vi "Menu.Simulate, Set Menu State.vi"(8 "error in (no error)":errorcluster, 9 "Sim Enable":bool, 10 "Menu Tag":string, 11 "Menu Ref":refnum<k9>) -> (0 "error out":errorcluster, 2 "Sim ON":bool)   [LabVIEW 2024, in "EQMF.lvlib" / "Menu Utils.lvlib"]
uses:
  Menu Utils.lvlib
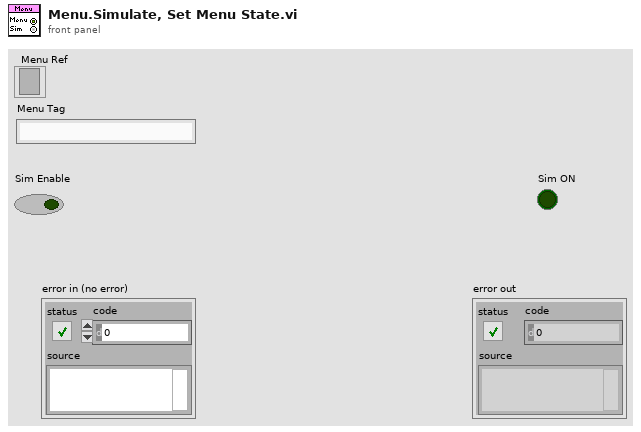
[diagram p1: front panel]
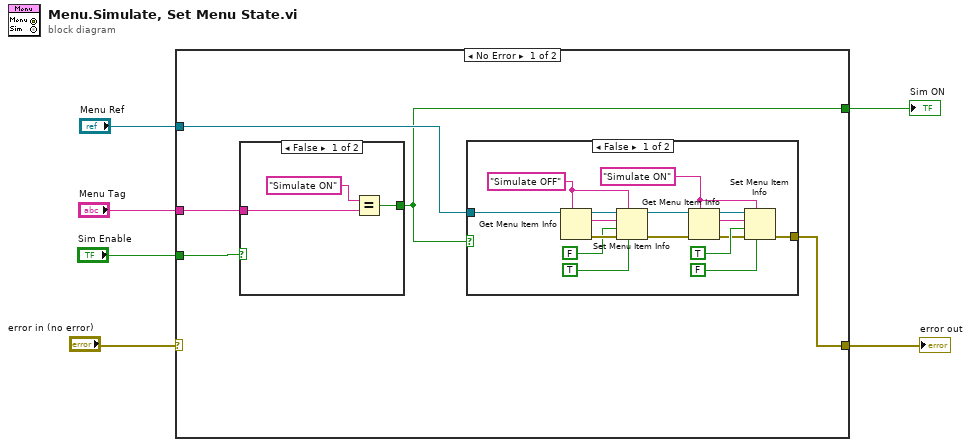
[diagram p0: block diagram]
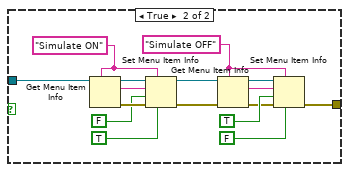
[diagram p3: hidden frame]
diagram:
  n1 = case shown="No Error" "error in (no error)" {
    selector: "error in (no error)" -> [_ w48]
    tunnel: "Menu Ref" -> [w11 _]
    tunnel: "Sim Enable" -> [w10 _]
    tunnel: "Menu Tag" -> [w9 _]
    tunnel: [w8 w48] -> w2
    tunnel: [w7 _] -> w1
    frame No Error {
      n2 = case shown="False" w10 {
        selector: w10 -> [_ w15]
        tunnel: w9 -> [w13 _]
        tunnel: [w12 w15] -> w7
        frame False {
          n3 = Equal?(x="Simulate ON", y=w13) -> (x = y?=w12:bool)
        }
        frame True {
        }
      }
      n4 = case shown="False" w7 {
        tunnel: w11 -> [w29 w45]
        tunnel: [w16 w32] -> w8
        frame False {
          w18 = "Simulate OFF"
          w20 = "Simulate ON"
          n5 = Get Menu Item Info(7:w18, 11:w29) -> (0:w30:errorcluster, 2:w28:string, 3:w31:refnum<k9>)  [unwired: 1 in, 4 out]
          n6 = Set Menu Item Info(6:TRUE, 7:w18, 8:w30, 9:FALSE, 10:w28, 11:w31) -> (0:w17:errorcluster, 3:w19:refnum<k9>)  [unwired: 1 in]
          n7 = Get Menu Item Info(7:w20, 8:w17, 11:w19) -> (0:w22:errorcluster, 2:w23:string, 3:w21:refnum<k9>)  [unwired: 4 out]
          n8 = Set Menu Item Info(6:FALSE, 7:w20, 8:w22, 9:TRUE, 10:w23, 11:w21) -> (0:w16:errorcluster)  [unwired: 1 in, 1 out]
        }
        frame True {
          w34 = "Simulate ON"
          w36 = "Simulate OFF"
          n9 = Get Menu Item Info(7:w34, 11:w45) -> (0:w46:errorcluster, 2:w44:string, 3:w47:refnum<k9>)  [unwired: 1 in, 4 out]
          n10 = Set Menu Item Info(6:TRUE, 7:w34, 8:w46, 9:FALSE, 10:w44, 11:w47) -> (0:w33:errorcluster, 3:w35:refnum<k9>)  [unwired: 1 in]
          n11 = Get Menu Item Info(7:w36, 8:w33, 11:w35) -> (0:w38:errorcluster, 2:w39:string, 3:w37:refnum<k9>)  [unwired: 4 out]
          n12 = Set Menu Item Info(6:FALSE, 7:w36, 8:w38, 9:TRUE, 10:w39, 11:w37) -> (0:w32:errorcluster)  [unwired: 1 in, 1 out]
        }
      }
    }
    frame Error {
    }
  }
  "error out" <- w2
  "Sim ON" <- w1
